vi "Read Scheduled.vi"(7 "scheduled time":timestamp, 10 "channel":T1) -> (1 "last element?":bool, 2 "element":T2, 3 "element valid?":bool, 5 "actual time":timestamp, 6 "count":i32)   [LabVIEW 2017, in "Stream-t'WPI_EncoderType.ctl'.lvlib"]
doc: "Reads an element from a Stream channel at a scheduled time. The endpoint waits if no element is available in the channel at the scheduled time."
uses:
  <extravilib>/ChannelInstances/Stream-t'WPI_EncoderType.ctl'.lvlib
  <vilib>/Rock Robotics/WPI/Encoder/WPI_EncoderType.ctl
  <extravilib>/ChannelInstances/Stream-t'WPI_EncoderType.ctl'/)Channel.ctl
  <extravilib>/ChannelInstances/Stream-t'WPI_EncoderType.ctl'/Read With Abort.vi
  <extravilib>/ChannelInstances/Stream-t'WPI_EncoderType.ctl'/EndpointRead.vi
  <resource>/ChannelSupport/_ChannelSupport/WaitIfNeeded.vi
  <extravilib>/ChannelInstances/Stream-t'WPI_EncoderType.ctl'/)Channel.vi
  <resource>/ChannelSupport/_ChannelSupport/_ChannelSupport.lvlib
  <resource>/ChannelSupport/_ChannelSupport/GetErrors/FpgaChannelWireNotSupported.xnode
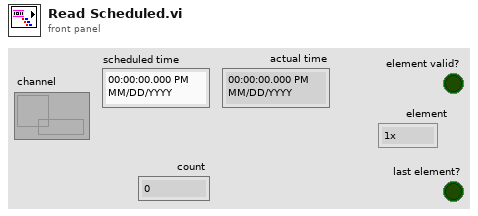
[diagram p1: front panel]
types:
  T1 = typedef "Stream-t'WPI_EncoderType.ctl'.lvlib/)Channel.ctl" = refnum<queue>
  T2 = typedef "WPI_EncoderType.ctl" = enum16{"1x", "2x", "4x"}
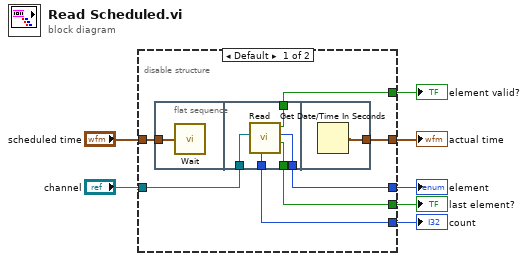
[diagram p0: block diagram]
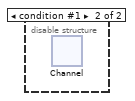
[diagram p2: hidden frame]
diagram:
  n1 = disable-structure shown="Default" {
    disable-tunnel: "scheduled time" -> [w14 _]
    disable-tunnel: [w13 _] -> w6
    disable-tunnel: "channel" -> [w12 _]
    disable-tunnel: [w11 _] -> w4
    disable-tunnel: [w10 _] -> w3
    disable-tunnel: [w9 _] -> w2
    disable-tunnel: [w8 _] -> w1
    frame condition #0 (active) {
      n2 = flat-sequence {
        tunnel: w14 -> [w15]
        tunnel: w12 -> [w20]
        tunnel: [w18] -> w11
        tunnel: [w19] -> w10
        tunnel: [w17] -> w9
        tunnel: [w16] -> w8
        tunnel: [w21] -> w13
        frame #0 {
          n3 = call <resource>:"Wait.vi"("desired time"=w15) -> ()  [unwired: 2 out]
        }
        frame #1 {
          n4 = call <extravilib>:"Read.vi"("channel"=w20) -> ("last element?"=w16:bool, "element"=w18:T2, "element valid?"=w17:bool, "count"=w19:i32)  [unwired: 6 in, 1 out]
        }
        frame #2 {
          n5 = Get Date/Time In Seconds() -> (seconds since 1Jan1904=w21:timestamp)
        }
      }
    }
    frame condition #1 {
      n6 = xnode "Channel"() -> ()
    }
  }
  "element" <- w4
  "actual time" <- w6
  "count" <- w3
  "element valid?" <- w2
  "last element?" <- w1
